vi "Create.vi"() -> (3 "Dictionary":variant)   [LabVIEW 2013, in "Dictionary.lvlib"]
doc: "Creates an empty dictionary."
uses:
  Dictionary.lvlib
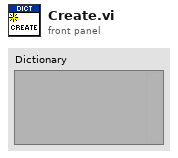
[diagram p1: front panel]
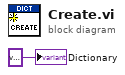
[diagram p0: block diagram]
diagram:
  "Dictionary" <- variant ("Dictionary")
